vi "cDAQ Get Temp Data.vi"(7 "Error In":errorcluster, 10 "Input Task":refnum<k21>) -> (0 "Error Out":errorcluster, 1 "Gas Temp":T1, 2 "Mean & StdDev":T1[](array[typedef]), 3 "Task Out":refnum<k21>, 4 "Measurements":dbl[][](array[numeric]) format="%0.2f", 5 "to cDAQ output":dbl[](array[numeric]))   [LabVIEW 2016]
doc: "TC data is read from cDAQ using NI Max. All configurations are done in NI Max. Multiple data points are acquired for each sensor and averaged (along with std dev.) These avg'd temp measurements are displayed in Panels 1-4. Temp is displayed as either in bounds (green) or out of bounds (red)."
uses:
  <vilib>/Analysis/NI_AALBase.lvlib
  Type Definitions/Instrument Sensor.ctl
  <vilib>/DAQmx/read.llb/DAQmx Read (Analog 2D DBL NChan NSamp).vi
  Type Definitions/TC Cluster Panel.ctl
  Type Definitions/Panel.ctl
panel:
  out "Voltages Graph":dbl[][](graph)
  in  "TC Min OK Val":dbl
  in  "TC Max OK Val":dbl
  in  "StDev Upper Limit":dbl
  in  "Panel 4: 55-72":i32[](array[numeric])=[16, 17, 18, 19, 20, 21, 22, 23, 24, 0, 0, 0, 0, 0, 0, 0, 7, 8]
  in  "Panel 3: 37-54":i32[](array[numeric])=[32, 33, 34, 35, 36, 37, 38, 39, 40, 41, 42, 0, 0, 0, 0, 0, 5, 6]
  in  "Panel 2: 19-36":i32[](array[numeric])=[48, 49, 50, 51, 52, 53, 54, 55, 56, 57, 58, 59, 60, 61, 62, 63, 3, 4]
  in  "Panel 1: 1-18":i32[](array[numeric])=[65, 66, 67, 68, 69, 0, 0, 0, 0, 0, 0, 0, 0, 0, 0, 0, 1, 2]
  in  "TC Cluster Panels":T2={"Panel 1"={"1"={"Mean"=0.0, " Std"=0.0, "Color Box"=0}, "2"={"Mean"=0.0, " Std"=-7.028284921808887e+221, "Color Box"=0}, "3"={"Mean"=0.0, " Std"=0.0, "Color Box"=0}, "4"={"Mean"=0.0, " Std"=0.0, "Color Box"=0}, "5"={"Mean"=0.0, " Std"=0.0, "Color Box"=0}, "6"={"Mean"=0.0, " Std"=0.0, "Color Box"=0}, "7"={"Mean"=0.0, " Std"=0.0, "Color Box"=0}, "8"={"Mean"=0.0, " Std"=0.0, "Color Box"=0}, "9"={"Mean"=0.0, " Std"=0.0, "Color Box"=0}, "10"={"Mean"=0.0, " Std"=0.0, "Color Box"=0}, "11"={"Mean"=0.0, " Std"=0.0, "Color Box"=0}, "12"={"Mean"=0.0, " Std"=0.0, "Color Box"=0}, "13"={"Mean"=0.0, " Std"=0.0, "Color Box"=0}, "14"={"Mean"=0.0, " Std"=0.0, "Color Box"=0}, "15"={"Mean"=0.0, " Std"=0.0, "Color Box"=0}, "16"={"Mean"=0.0, " Std"=0.0, "Color Box"=0}, "17"={"Mean"=0.0, " Std"=0.0, "Color Box"=0}, "18"={"Mean"=0.0, " Std"=0.0, "Color Box"=0}}, "Panel 2"={"1"={"Mean"=0.0, " Std"=0.0, "Color Box"=0}, "2"={"Mean"=0.0, " Std"=4.1433337045841466e-94, "Color Box"=0}, "3"={"Mean"=0.0, " Std"=0.0, "Color Box"=0}, "4"={"Mean"=0.0, " Std"=0.0, "Color Box"=0}, "5"={"Mean"=0.0, " Std"=0.0, "Color Box"=0}, "6"={"Mean"=0.0, " Std"=0.0, "Color Box"=0}, "7"={"Mean"=0.0, " Std"=0.0, "Color Box"=0}, "8"={"Mean"=0.0, " Std"=0.0, "Color Box"=0}, "9"={"Mean"=0.0, " Std"=0.0, "Color Box"=0}, "10"={"Mean"=0.0, " Std"=0.0, "Color Box"=0}, "11"={"Mean"=0.0, " Std"=0.0, "Color Box"=0}, "12"={"Mean"=0.0, " Std"=0.0, "Color Box"=0}, "13"={"Mean"=0.0, " Std"=0.0, "Color Box"=0}, "14"={"Mean"=0.0, " Std"=0.0, "Color Box"=0}, "15"={"Mean"=0.0, " Std"=0.0, "Color Box"=0}, "16"={"Mean"=0.0, " Std"=0.0, "Color Box"=0}, "17"={"Mean"=0.0, " Std"=0.0, "Color Box"=0}, "18"={"Mean"=0.0, " Std"=0.0, "Color Box"=0}}, "Panel 3"={"1"={"Mean"=0.0, " Std"=0.0, "Color Box"=0}, "2"={"Mean"=0.0, " Std"=-6.5270924912614764e+221, "Color Box"=0}, "3"={"Mean"=0.0, " Std"=0.0, "Color Box"=0}, "4"={"Mean"=0.0, " Std"=0.0, "Color Box"=0}, "5"={"Mean"=0.0, " Std"=0.0, "Color Box"=0}, "6"={"Mean"=0.0, " Std"=0.0, "Color Box"=0}, "7"={"Mean"=0.0, " Std"=0.0, "Color Box"=0}, "8"={"Mean"=0.0, " Std"=0.0, "Color Box"=0}, "9"={"Mean"=0.0, " Std"=0.0, "Color Box"=0}, "10"={"Mean"=0.0, " Std"=0.0, "Color Box"=0}, "11"={"Mean"=0.0, " Std"=0.0, "Color Box"=0}, "12"={"Mean"=0.0, " Std"=0.0, "Color Box"=0}, "13"={"Mean"=0.0, " Std"=0.0, "Color Box"=0}, "14"={"Mean"=0.0, " Std"=0.0, "Color Box"=0}, "15"={"Mean"=0.0, " Std"=0.0, "Color Box"=0}, "16"={"Mean"=0.0, " Std"=0.0, "Color Box"=0}, "17"={"Mean"=0.0, " Std"=0.0, "Color Box"=0}, "18"={"Mean"=0.0, " Std"=0.0, "Color Box"=0}}, "Panel 4"={"1"={"Mean"=0.0, " Std"=0.0, "Color Box"=0}, "2"={"Mean"=0.0, " Std"=2.1824123077342332e+252, "Color Box"=0}, "3"={"Mean"=0.0, " Std"=0.0, "Color Box"=0}, "4"={"Mean"=0.0, " Std"=0.0, "Color Box"=0}, "5"={"Mean"=0.0, " Std"=0.0, "Color Box"=0}, "6"={"Mean"=0.0, " Std"=0.0, "Color Box"=0}, "7"={"Mean"=0.0, " Std"=0.0, "Color Box"=0}, "8"={"Mean"=0.0, " Std"=0.0, "Color Box"=0}, "9"={"Mean"=0.0, " Std"=0.0, "Color Box"=0}, "10"={"Mean"=0.0, " Std"=0.0, "Color Box"=0}, "11"={"Mean"=0.0, " Std"=0.0, "Color Box"=0}, "12"={"Mean"=0.0, " Std"=0.0, "Color Box"=0}, "13"={"Mean"=0.0, " Std"=0.0, "Color Box"=0}, "14"={"Mean"=0.0, " Std"=0.0, "Color Box"=0}, "15"={"Mean"=0.0, " Std"=0.0, "Color Box"=0}, "16"={"Mean"=0.0, " Std"=0.0, "Color Box"=0}, "17"={"Mean"=0.0, " Std"=0.0, "Color Box"=0}, "18"={"Mean"=0.0, " Std"=0.0, "Color Box"=0}}}
  # "NI Max Physical Channel Index"
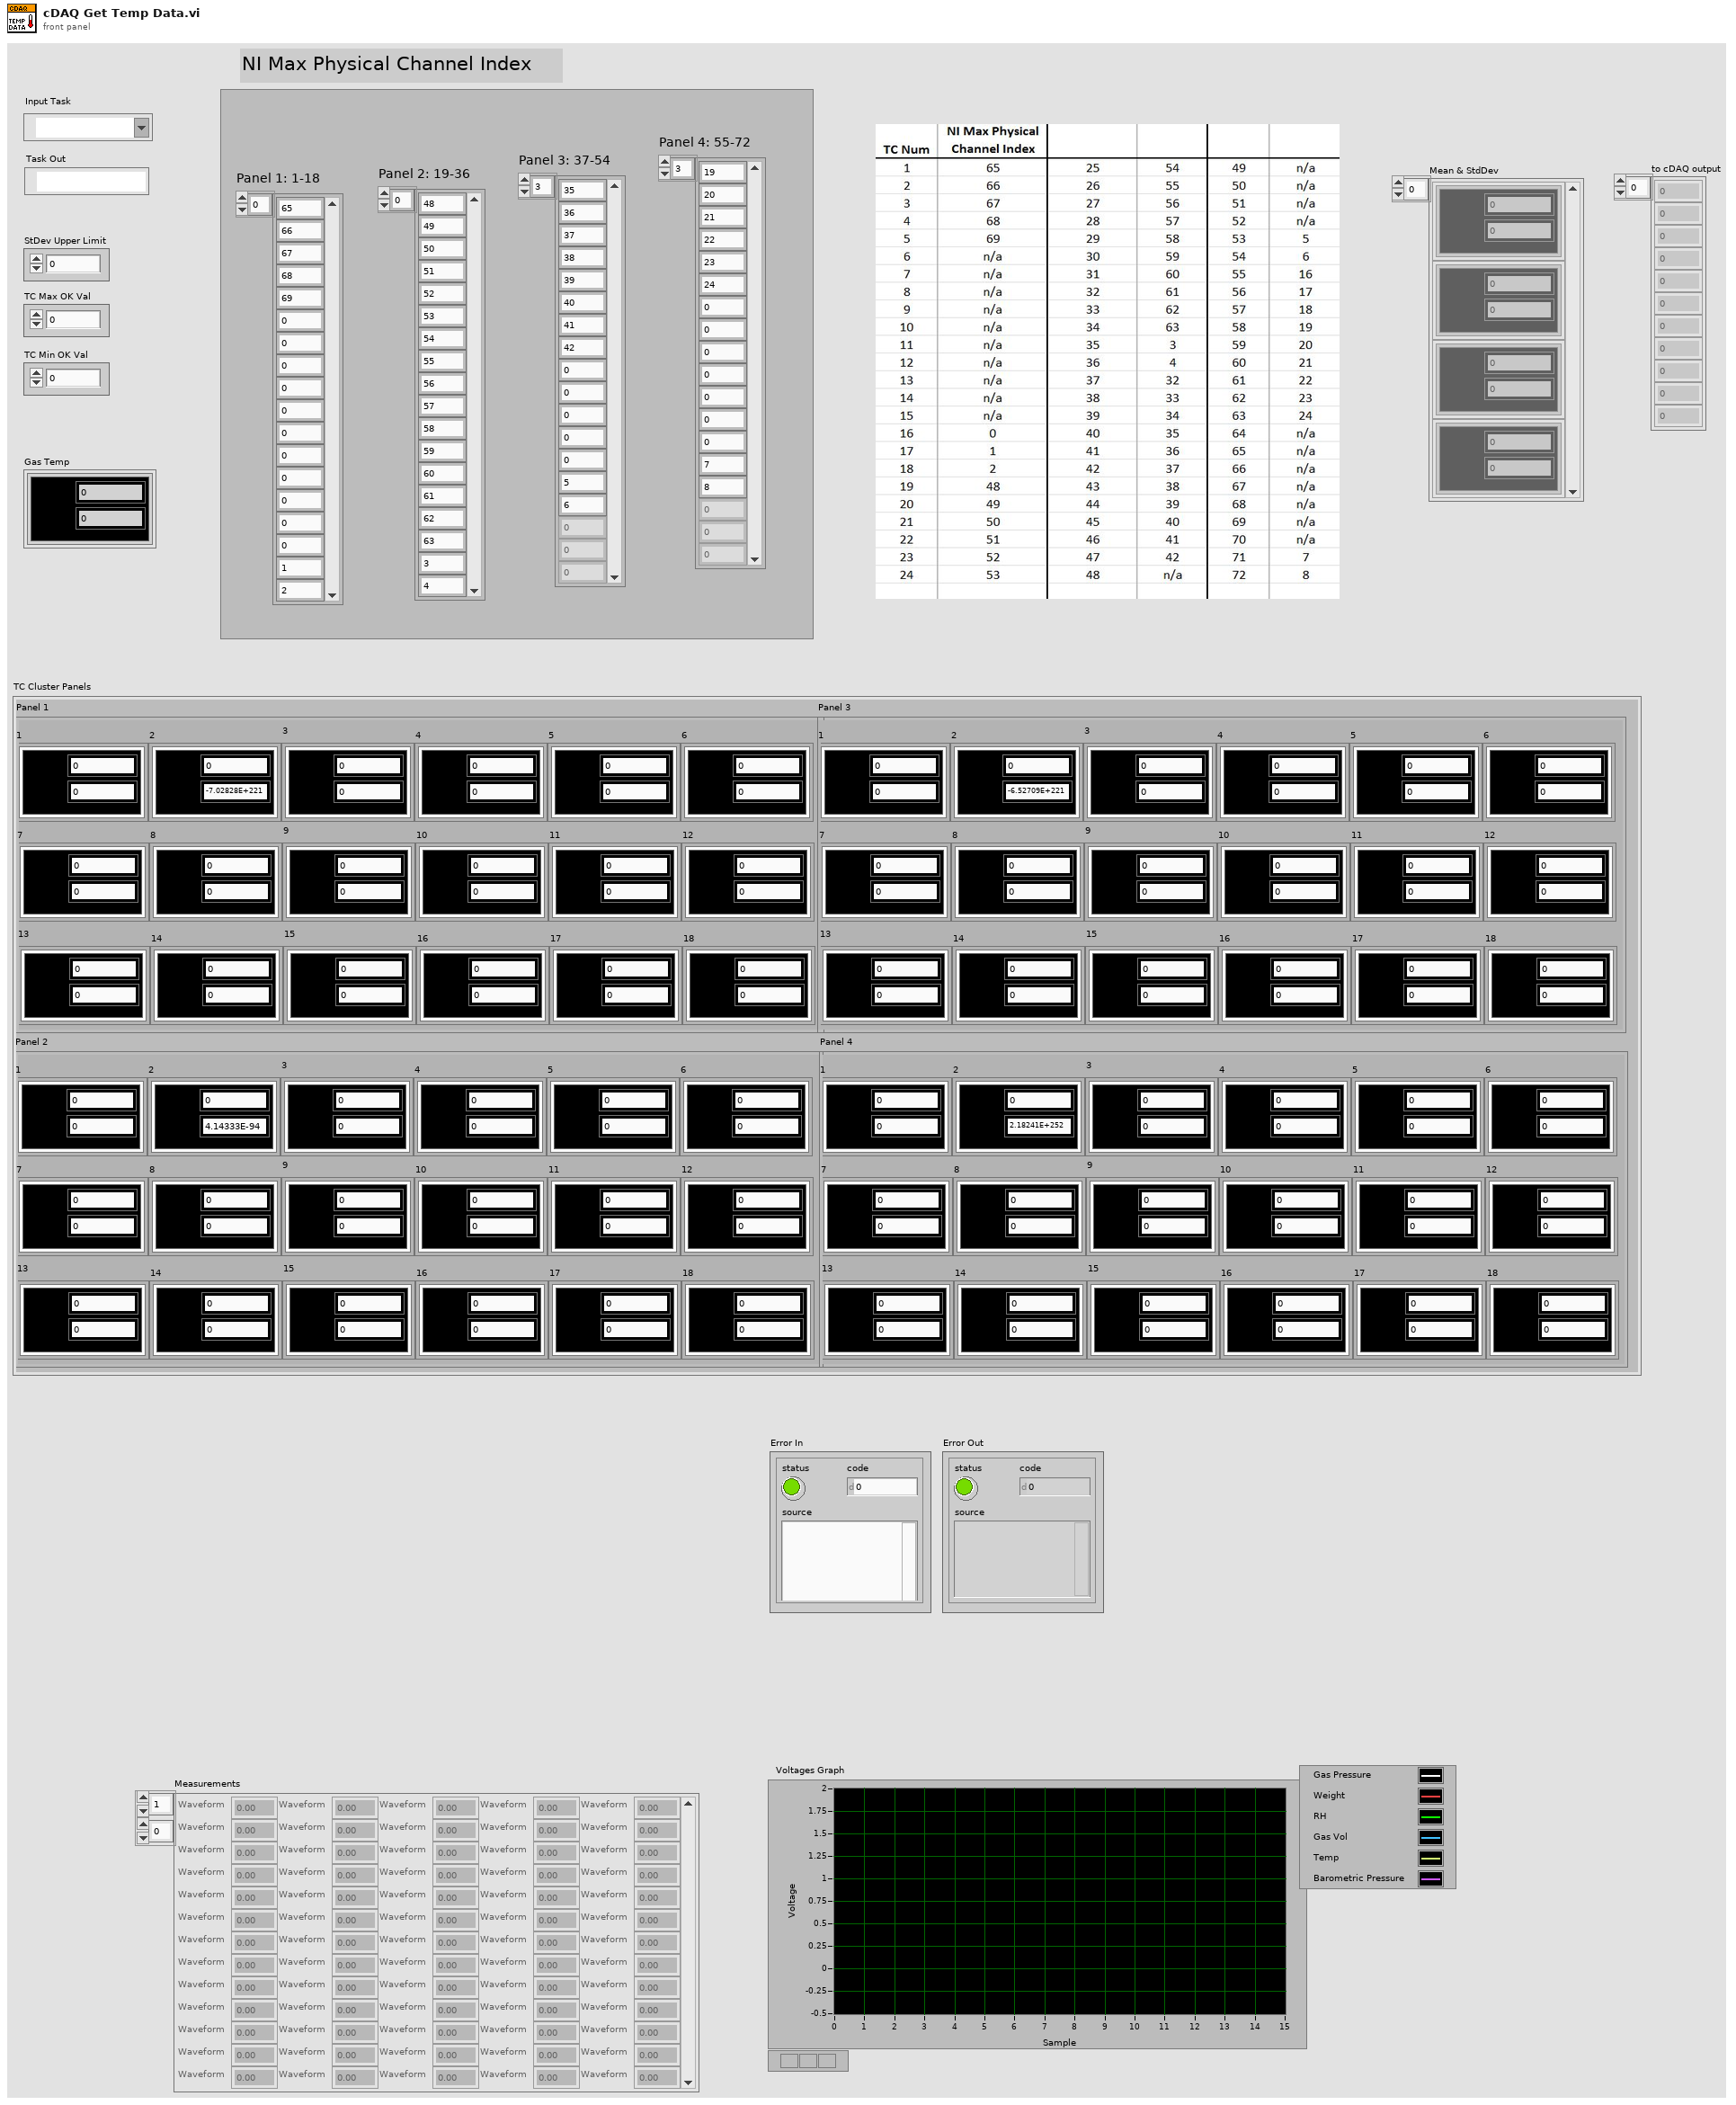
[diagram p1: front panel]
types:
  T1 = typedef "Instrument Sensor.ctl" = cluster{"Mean":dbl, " Std":dbl, "Color Box":u32}
  T2 = typedef "TC Cluster Panel.ctl" = cluster{"Panel 1":T3, "Panel 2":T3, "Panel 3":T3, "Panel 4":T3}
  T3 = typedef "Panel.ctl" = cluster{"1":T1, "2":T1, "3":T1, "4":T1, "5":T1, "6":T1, "7":T1, "8":T1, "9":T1, "10":T1, "11":T1, "12":T1, "13":T1, "14":T1, "15":T1, "16":T1, "17":T1, "18":T1}
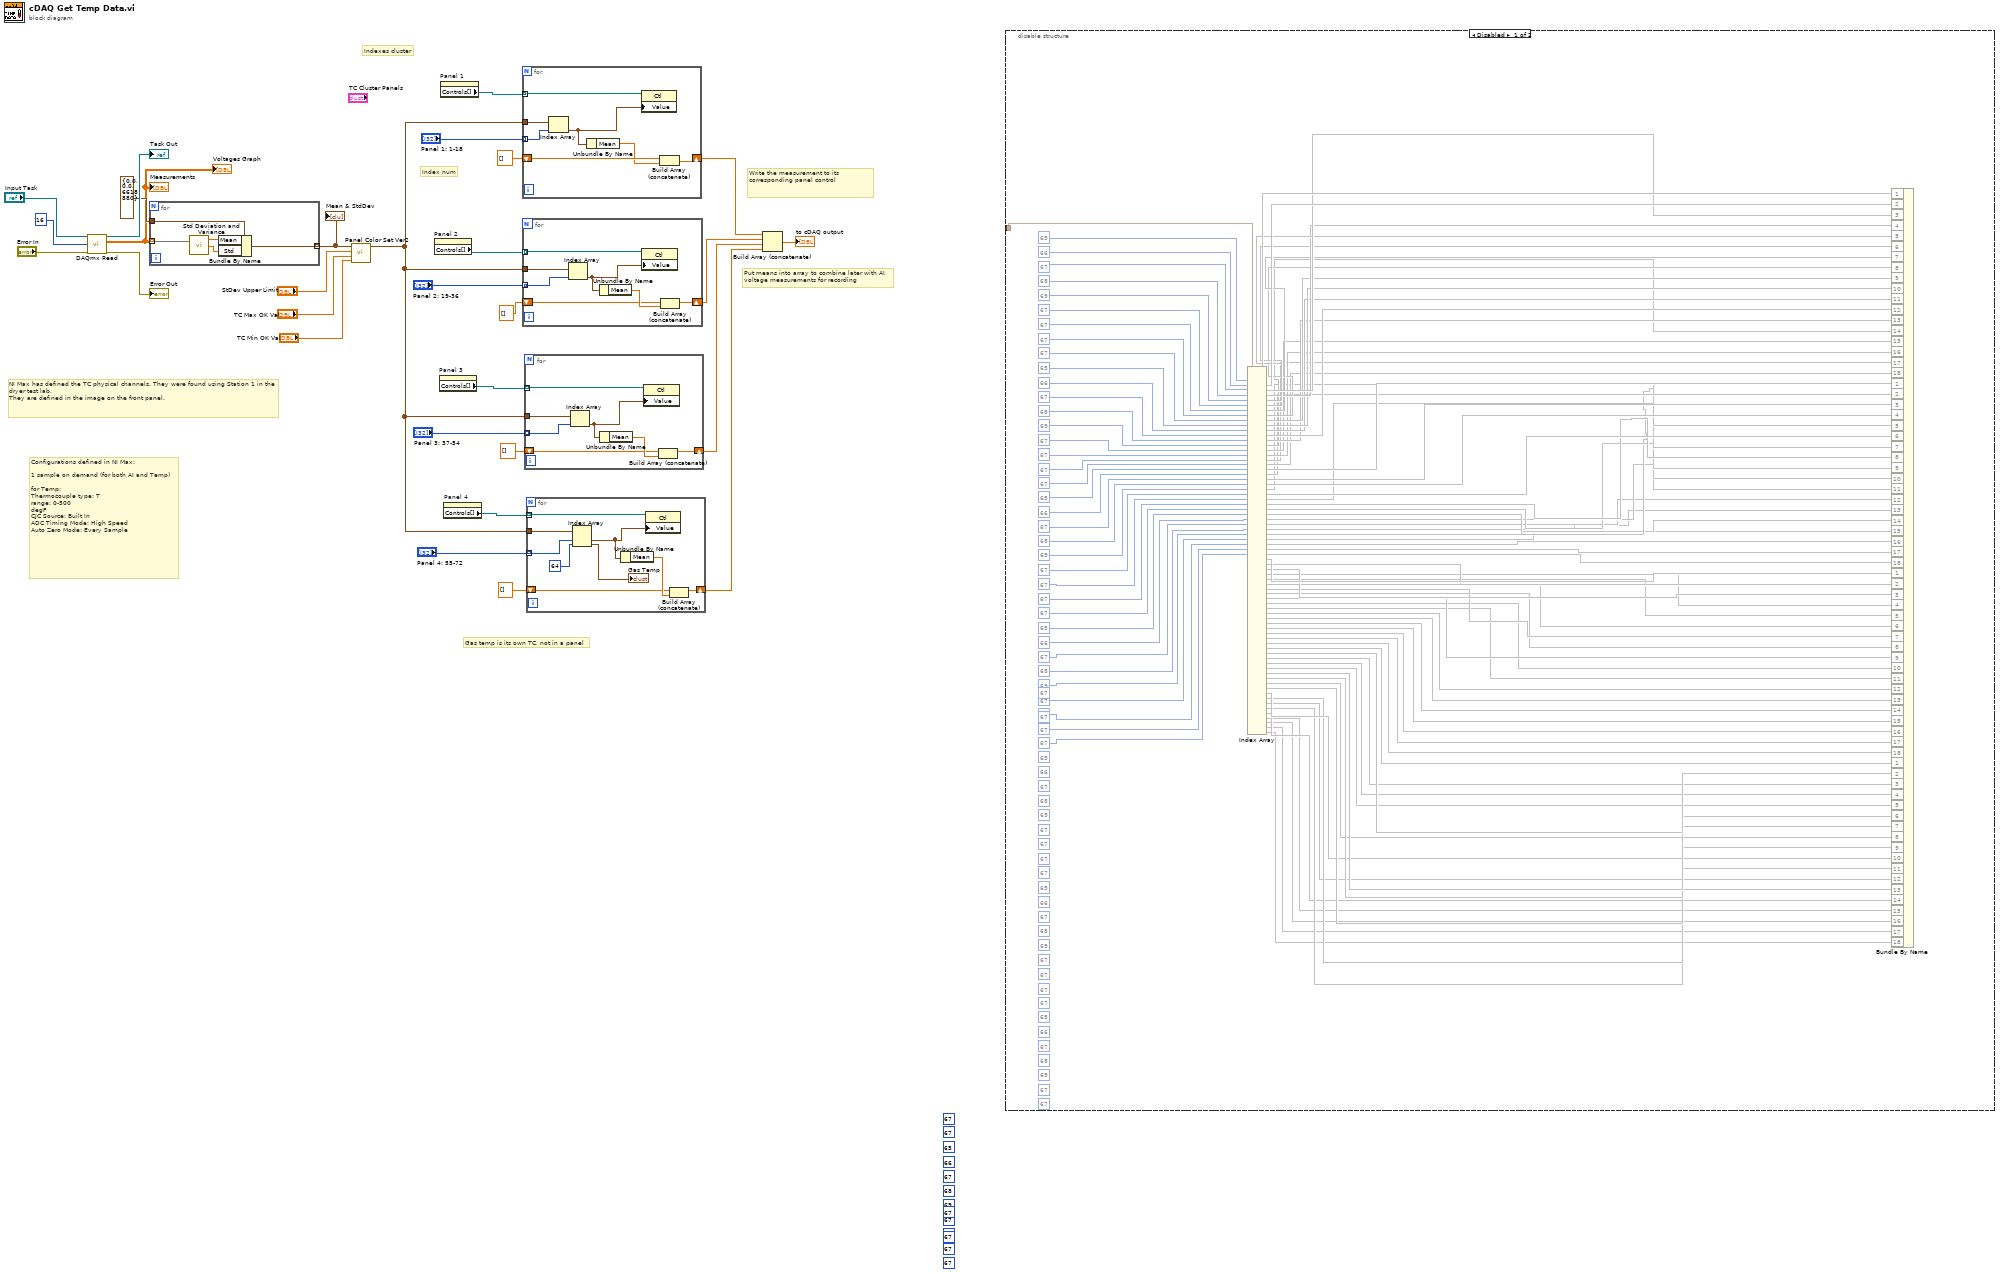
[diagram p0: block diagram]
diagram:
  (unwired) 67 ("index")
  (unwired) 67 ("index")
  (unwired) 67 ("index")
  (unwired) 67 ("index")
  (unwired) 69 ("index")
  (unwired) 68 ("index")
  (unwired) 67 ("index")
  (unwired) 66 ("index")
  (unwired) 65 ("index (row)")
  (unwired) 67 ("index")
  (unwired) 67 ("index")
  (unwired) 67 ("index")
  (unwired) 67 ("index")
  # "Put means into array to combine later with AI\nvoltage measurements for recording"
  # "Write the measurement to its corresponding panel control"
  # "Gas temp is its own TC, not in a panel"
  # "Index num"
  # "Configurations defined in NI Max:\n \n1 sample on demand (for both AI and Temp)\n\nfor Temp: \nThermocouple type: T\nrange: 0-500\ndegF\nCJC Source: Built In\nADC Timing Mode: High Speed\nAuto Zero Mode: Every Sample"
  # "Indexes cluster"
  # "NI Max has defined the TC physical channels. They were found using Station 1 in the dryer test lab.\nThey are defined in the image on the front panel."
  n1 = call-poly <vilib>:"DAQmx Read.vi"("task/channels in"="Input Task", "number of samples per channel"=16, "error in"="Error In") -> ("task out"=→"Task Out":refnum<k21>, "data"=w10:dbl[][], "error out"=→"Error Out":errorcluster)  [unwired: 10 in]
  "Measurements" <- w10
  "Voltages Graph" <- w10
  n2 = for {
    tunnel: w10 -> [w34] mode=indexing
    tunnel: [w31] -> w11 mode=indexing
    tunnel: T1 {"Mean"=0.0, " Std"=0.0, "Color Box"=6618880} ("cluster") -> [w30]
    n3 = call <vilib>:"Std Deviation and Variance.vi"("X"=w34) -> ("mean"=w33:dbl, "standard deviation"=w32:dbl)  [unwired: 1 in, 1 out]
    n4 = Bundle By Name(cluster=w30, "Mean"=w33, "Std"=w32) -> (w31:T1)
  }
  "Mean & StdDev" <- w11
  n5 = call "Panel Color Set Ver2.vi"("TC Min OK Val"="TC Min OK Val", "TC Max OK Val"="TC Max OK Val", "StDev Thresh"="StDev Upper Limit", "Input Block"=w11) -> ("Output Block"=w21:T1[])  [unwired: 2 in]
  n6 = property on="Panel 2" class="Clust (strict)"() -> ("Controls[]"=w24:refnum<vi>[])  [unwired: 2 in, 2 out]
  n7 = property on="Panel 3" class="Clust (strict)"() -> ("Controls[]"=w23:refnum<vi>[])  [unwired: 2 in, 2 out]
  n8 = property on="Panel 1" class="Clust (strict)"() -> ("Controls[]"=w25:refnum<vi>[])  [unwired: 2 in, 2 out]
  n9 = property on="Panel 4" class="Clust (strict)"() -> ("Controls[]"=w22:refnum<vi>[])  [unwired: 2 in, 2 out]
  n10 = for {
    tunnel: w25 -> [w41] mode=indexing
    tunnel: w21 -> [w40]
    tunnel: "Panel 1: 1-18" -> [w39] mode=indexing
    shift-right: [w35] -> w8
    shift-left: dbl[] [] -> [w37]
    n11 = Index Array(array=w40, index=w39) -> (element=w38:T1)
    n12 = Unbundle By Name(w38) -> ("Mean"=w36:dbl)
    n13 = property class="Ctl"(reference=w41, "Value"=w38) -> ()  [unwired: 1 in, 2 out]
    n14 = Build Array (concatenate)(w37, w36) -> (w35:dbl[])
  }
  n15 = for {
    tunnel: w24 -> [w48] mode=indexing
    tunnel: w21 -> [w47]
    tunnel: "Panel 2: 19-36" -> [w46] mode=indexing
    shift-right: [w42] -> w4
    shift-left: dbl[] [] -> [w44]
    n16 = Index Array(array=w47, index=w46) -> (element=w43:T1)
    n17 = Unbundle By Name(w43) -> ("Mean"=w45:dbl)
    n18 = property class="Ctl"(reference=w48, "Value"=w43) -> ()  [unwired: 1 in, 2 out]
    n19 = Build Array (concatenate)(w44, w45) -> (w42:dbl[])
  }
  n20 = for {
    tunnel: w23 -> [w55] mode=indexing
    tunnel: w21 -> [w54]
    tunnel: "Panel 3: 37-54" -> [w53] mode=indexing
    shift-right: [w50] -> w3
    shift-left: dbl[] [] -> [w51]
    n21 = Index Array(array=w54, index=w53) -> (element=w49:T1)
    n22 = Unbundle By Name(w49) -> ("Mean"=w52:dbl)
    n23 = property class="Ctl"(reference=w55, "Value"=w49) -> ()  [unwired: 1 in, 2 out]
    n24 = Build Array (concatenate)(w51, w52) -> (w50:dbl[])
  }
  n25 = for {
    tunnel: w22 -> [w64] mode=indexing
    tunnel: w21 -> [w63]
    tunnel: "Panel 4: 55-72" -> [w62] mode=indexing
    shift-right: [w57] -> w2
    shift-left: dbl[] [] -> [w58]
    n26 = Index Array(array=w63, index #1=w62, index #2=64 ("index")) -> (element #1=w56:T1, element #2=→"Gas Temp":T1)
    n27 = Unbundle By Name(w56) -> ("Mean"=w59:dbl)
    n28 = property class="Ctl"(reference=w64, "Value"=w56) -> ()  [unwired: 1 in, 2 out]
    n29 = Build Array (concatenate)(w58, w59) -> (w57:dbl[])
  }
  n30 = Build Array (concatenate)(w8, w4, w3, w2) -> (→"to cDAQ output":dbl[])
  n31 = disable-structure shown="Disabled" {
    disable-tunnel: _ -> [w65 _]
    frame Disabled {
      (unwired) 67 ("index")
      (unwired) 67 ("index")
      (unwired) 69 ("index")
      (unwired) 68 ("index")
      (unwired) 67 ("index")
      (unwired) 66 ("index")
      (unwired) 65 ("index (row)")
      (unwired) 67 ("index")
      (unwired) 67 ("index")
      (unwired) 67 ("index")
      (unwired) 67 ("index")
      (unwired) 69 ("index")
      (unwired) 68 ("index")
      (unwired) 67 ("index")
      (unwired) 66 ("index")
      (unwired) 65 ("index (row)")
      (unwired) 67 ("index")
      (unwired) 67 ("index")
      (unwired) 67 ("index")
      (unwired) 67 ("index")
      (unwired) 69 ("index")
      (unwired) 68 ("index")
      (unwired) 67 ("index")
      (unwired) 66 ("index")
      (unwired) 65 ("index (row)")
      (unwired) 67 ("index")
      (unwired) 67 ("index")
      n32 = Index Array(array=w65, index #1=65 ("index (row)"), index #2=66 ("index"), index #3=67 ("index"), index #4=68 ("index"), index #5=69 ("index"), index #6=67 ("index"), index #7=67 ("index"), index #8=67 ("index"), index #9=67 ("index"), index #10=65 ("index (row)"), index #11=66 ("index"), index #12=67 ("index"), index #13=68 ("index"), index #14=69 ("index"), index #15=67 ("index"), index #16=67 ("index"), index #17=67 ("index"), index #18=67 ("index"), index #19=65 ("index (row)"), index #20=66 ("index"), index #21=67 ("index"), index #22=68 ("index"), index #23=69 ("index"), index #24=67 ("index"), index #25=67 ("index"), index #26=67 ("index"), index #27=67 ("index"), index #28=65 ("index (row)"), index #29=66 ("index"), index #30=67 ("index"), index #31=68 ("index"), index #32=69 ("index"), index #33=67 ("index"), index #34=67 ("index"), index #35=67 ("index"), index #36=67 ("index")) -> (element #1=w172, element #2=w171, element #3=w170, element #4=w165, element #5=w166, element #6=w164, element #7=w163, element #8=w162, element #9=w161, element #10=w160, element #11=w159, element #12=w158, element #13=w157, element #14=w156, element #15=w155, element #16=w154, element #17=w153, element #18=w152, element #19=w151, element #20=w150, element #21=w149, element #22=w148, element #23=w147, element #24=w146, element #25=w145, element #26=w144, element #27=w143, element #28=w142, element #29=w141, element #30=w140, element #31=w139, element #32=w138, element #33=w137, element #34=w136, element #35=w135, element #36=w134, element #37=w133, element #38=w132, element #39=w131, element #40=w130, element #41=w129, element #42=w128, element #43=w127, element #44=w126, element #45=w125, element #46=w124, element #47=w123, element #48=w122, element #49=w121, element #50=w120, element #51=w119, element #52=w118, element #53=w117, element #54=w116, element #55=w115, element #56=w114, element #57=w113, element #58=w112, element #59=w111, element #60=w110, element #61=w109, element #62=w108, element #63=w107, element #64=w106, element #65=w105, element #66=w104, element #67=w103, element #68=w102, element #69=w101, element #70=w100, element #71=w99, element #72=w98)  [unwired: 36 in]
      n33 = Bundle By Name("1"=w172, "2"=w171, "3"=w170, "4"=w165, "5"=w166, "6"=w164, "7"=w163, "8"=w162, "9"=w161, "10"=w160, "11"=w159, "12"=w158, "13"=w157, "14"=w156, "15"=w155, "16"=w154, "17"=w153, "18"=w152, "1"=w151, "2"=w150, "3"=w149, "4"=w148, "5"=w147, "6"=w146, "7"=w145, "8"=w144, "9"=w143, "10"=w142, "11"=w141, "12"=w140, "13"=w139, "14"=w138, "15"=w137, "16"=w136, "17"=w135, "18"=w134, "1"=w133, "2"=w132, "3"=w131, "4"=w130, "5"=w129, "6"=w128, "7"=w127, "8"=w126, "9"=w125, "10"=w124, "11"=w123, "12"=w122, "13"=w121, "14"=w120, "15"=w119, "16"=w118, "17"=w117, "18"=w116, "1"=w115, "2"=w114, "3"=w113, "4"=w112, "5"=w111, "6"=w110, "7"=w109, "8"=w108, "9"=w107, "10"=w106, "11"=w105, "12"=w104, "13"=w103, "14"=w102, "15"=w101, "16"=w100, "17"=w99, "18"=w98) -> (w173:cluster{})  [unwired: 1 out]
    }
    frame Enabled {
    }
  }
